vi "empty task properties test.vi"() -> ()   [LabVIEW 2013]
uses:
  <resource>/objmgr/daqmx.rc
panel:
  out "Done":bool
  out "NumChans":u32
  out "Name":refnum<k21>
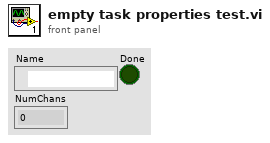
[diagram p1: front panel]
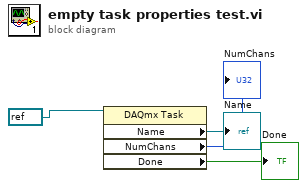
[diagram p0: block diagram]
diagram:
  n1 = property class="DAQmx Task"(reference=refnum<k21> refnum ("y")) -> ("Name"=→"Name":refnum<k21>, "NumChans"=→"NumChans":u32, "Done"=→"Done":bool)  [unwired: 1 in, 2 out]
